vi "TestGetCamFramesSimple.vi"() -> ()   [LabVIEW 2019]
panel:
  out "Intensity Graph":u16[][](graph)
  out "Array":u16[][](array[numeric])
  in  "FramesPerTrigger":u32
  out "size(s)":i32[](array[numeric])
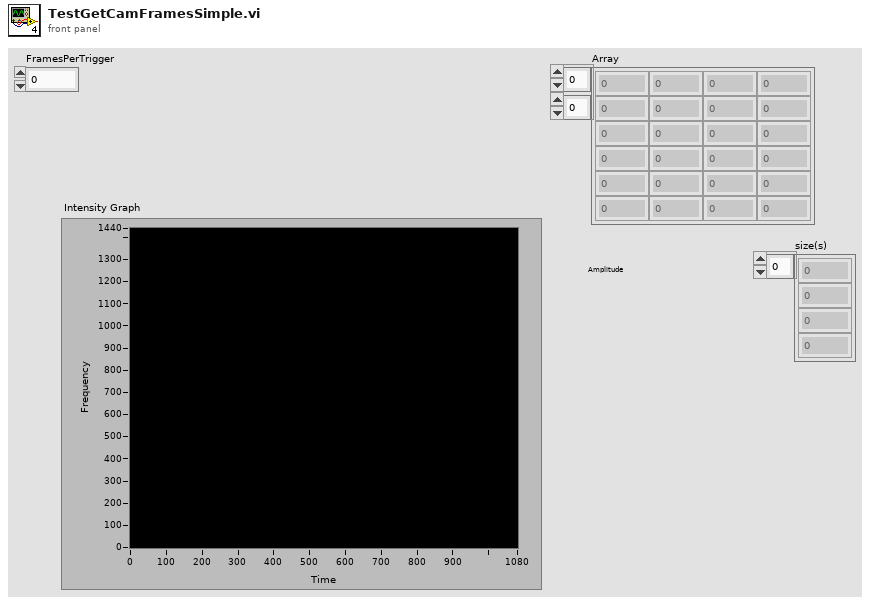
[diagram p1: front panel]
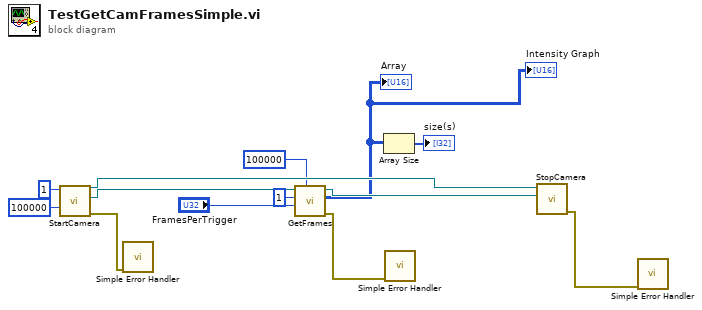
[diagram p0: block diagram]
diagram:
  n1 = call "StartCamera.vi"("ExposureTime_us"=u32 100000, "Gain"=u32 1) -> ("Error Out"=w5:errorcluster, "TLCamera reference out"=w13:refnum<k24>, "TLCameraSDK reference out"=w11:refnum<k24>)  [unwired: 7 in]
  n2 = call <vilib>:"Simple Error Handler.vi"("error in (no error)"=w5) -> ()  [unwired: 4 in, 5 out]
  n3 = call "GetFrames.vi"("ExposureTime_us"=u32 100000, "FramesPerTrigger"="FramesPerTrigger", "Gain"=u32 1, "TLCamera reference in"=w13) -> ("Error Out"=w4:errorcluster, "Array"=w1:u16[][], "TLCamera reference out"=w12:refnum<k24>)  [unwired: 5 in]
  "Array" <- w1
  "Intensity Graph" <- w1
  n4 = Array Size(array=w1) -> (size(s)=→"size(s)":i32[])
  n5 = call <vilib>:"Simple Error Handler.vi"("error in (no error)"=w4) -> ()  [unwired: 4 in, 5 out]
  n6 = call "StopCamera.vi"("TLCamera reference"=w12, "TLCameraSDK reference"=w11) -> ("Error Out"=w3:errorcluster)  [unwired: 9 in]
  n7 = call <vilib>:"Simple Error Handler.vi"("error in (no error)"=w3) -> ()  [unwired: 4 in, 5 out]
